vi "PH_Stepmotor_BaseClass.read Database.vi"(3 "error in (no error)":errorcluster, 5 "DB Entry to read":string) -> (0 "error out":errorcluster, 1 "Entry empty?":bool[](array[boolean]), 2 "Axes Data":cluster{"Axis_Scale":T1, "Endswitch?":bool}[](array[cluster]))   [LabVIEW 2014, in "PH_Stepmotor_BaseClass.lvlib"]
uses:
  PH_Stepmotor_BaseClass.lvlib
  PH_Stepmotor_BaseClass.Axis Settings.ctl
  PH_Stepmotor_BaseClass.Motor Type.ctl
  PH_Common/PH_Common.lvlib
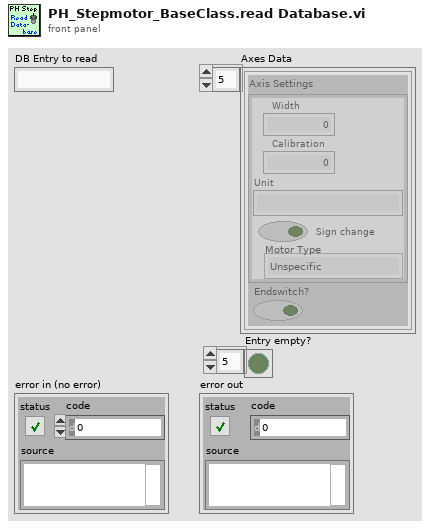
[diagram p1: front panel]
types:
  T1 = typedef "PH_Stepmotor_BaseClass.lvlib/PH_Stepmotor_BaseClass.Axis Settings.ctl" = cluster{"Sign change":bool, "Width":dbl, "Calibration":dbl, "Unit":string, "Motor Type":T2, "Unit Width":string, "Unit CF":string}
  T2 = typedef "PH_Stepmotor_BaseClass.lvlib/PH_Stepmotor_BaseClass.Motor Type.ctl" = enum16{"Unspecific", "OWIS 49.120.2633", "OWIS 49.060.1033", "OWIS 43.040.2558", "Diamond Motion 2200 series", "OWIS 49.120.266B.MV6", "Calorimeter", "Linear Stage 1", "MICOS VT-80", "MICOS VT-80 S", "Standa Rotstage nt0.95A", "PUF RA 320.200", "PUF RA 800.200", "PUF RA 800.400", "PUF RA 400.50", "1324.nn.800.50", "1324.n9c.800.50", "1324.nn.320.200", "1324.nn.400.200", "1324.nn.800.200", "1324.nn.400.50", "1324.8c9c.800.50", "1324.8c9c.400.200"}
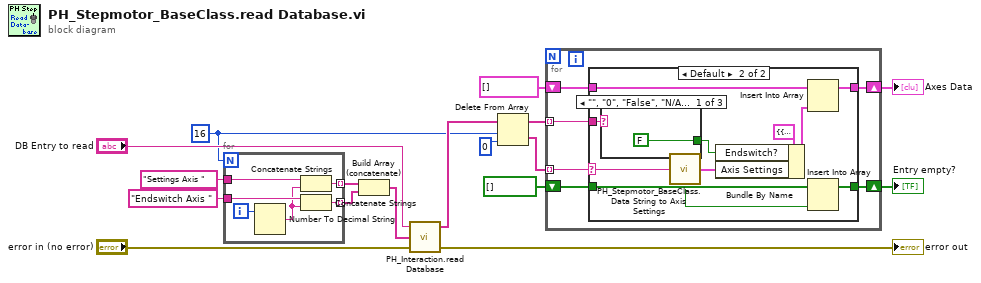
[diagram p0: block diagram]
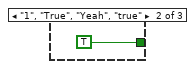
[diagram p3: hidden frame]
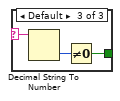
[diagram p4: hidden frame]
diagram:
  w1 = 16
  n1 = for {
    N: w1 -> [_]
    tunnel: "Settings Axis " -> [w22]
    tunnel: "Endswitch Axis " -> [w21]
    tunnel: [w19] -> w10 mode=indexing
    tunnel: [w18] -> w9 mode=indexing
    i -> [w23]
    n2 = Number To Decimal String(number=w23) -> (decimal integer string=w20:string)  [unwired: 1 in]
    n3 = Concatenate Strings(w22, w20) -> (w18:string)
    n4 = Concatenate Strings(w21, w20) -> (w19:string)
  }
  n5 = Build Array (concatenate)(w9, w10) -> (w11:string[])
  n6 = call "PH_Interaction.read Database.vi"("error in (no error)"="error in (no error)", "Strings to search for"=w11, "DB Entry to read"="DB Entry to read") -> ("error out"=→"error out":errorcluster, "Values"=w13:string[])  [unwired: 1 in]
  n7 = Delete From Array(array=w13, length=w1, index=0) -> (deleted portion=w14:string[], array with subset deleted=w15:string[])
  n8 = for {
    tunnel: w14 -> [w26] mode=indexing
    tunnel: w15 -> [w29] mode=indexing
    shift-right: [w27] -> w17
    shift-left: cluster{"Axis_Scale":T1, "Endswitch?":bool}[] [] ("Axes Data") -> [w28]
    shift-right: [w25] -> w3
    shift-left: bool[] [] -> [w24]
    n9 = case shown="Default" w26 {
      selector: w26 -> [_ w33]
      tunnel: w29 -> [_ w42]
      tunnel: w28 -> [w31 w41]
      tunnel: [w31 w40] -> w27
      tunnel: [w30 w35] -> w25
      tunnel: w24 -> [w30 w34]
      frame "N/A" {
      }
      frame Default {
        n10 = case shown="\"\", \"0\", \"False\", \"N/A\", \"None\", \"false\", \"no\", \"none\"" w42 {
          selector: w42 -> [_ _ w47]
          tunnel: [FALSE TRUE w45] -> w36
          frame "", "0", "False", "N/A", "None", "false", "no", "none" {
          }
          frame "1", "True", "Yeah", "true" {
          }
          frame Default {
            n11 = Decimal String To Number(string=w47) -> (number=w46:i32)  [unwired: 2 in, 1 out]
            n12 = Not Equal To 0?(x=w46) -> (x != 0?=w45:bool)
          }
        }
        n13 = call "PH_Stepmotor_BaseClass.Data String to Axis Settings.vi"("Data String"=w33) -> ("No axis"=w32:bool, "Axis Settings"=w37:T1)
        n14 = Bundle By Name(cluster=cluster{"Axis Settings":T1, "Endswitch?":bool} {"Axis Settings"={"Sign change"=FALSE, "Width"=0.0, "Calibration"=0.0, "Unit"="", "Motor Type"=enum."Unspecific", "Unit Width"="", "Unit CF"=""}, "Endswitch?"=FALSE} ("Axis Dataset"), "Endswitch?"=w36, "Axis Settings"=w37) -> (w38:cluster{"Axis Settings":T1, "Endswitch?":bool})
        n15 = Insert Into Array(array=w41, new element=w38) -> (w40:cluster{"Axis_Scale":T1, "Endswitch?":bool}[])  [unwired: 1 in]
        n16 = Insert Into Array(array=w34, new element=w32) -> (w35:bool[])  [unwired: 1 in]
      }
    }
  }
  "Axes Data" <- w17
  "Entry empty?" <- w3
